vi "SECoP_dataCreateSECoPstatus.vi"(8 "error in (no error)":errorcluster, 11 "DLL path (in)":T2) -> (0 "error out":errorcluster, 2 "SECoP_dataPtr (out)":T1 {"ptr64" format="%.0x"; "ptr32" format="%.0x"}, 3 "DLL path (out)":T2)   [LabVIEW 2023, in "SECoP.lvlib"]
doc: "Call <b>\"SECoP_dataCreateSECoPstatus.vi\"</b> to create a basic data type for a SECoP status with IDLE/100 only. Use <b>\"SECoP_dataPutEnumeration.vi\"</b> to extend it. Free resources after use with <b>\"SECoP_dataDestroy.vi\"</b>.\nNote: You could also use </b>\"SECoP-addStatusParameter.vi\"</b> to get a similar result.\n\n<b>DLL path</b> input and output of cluster from \"SECoP-Initialize.vi\"\n<b>SECoP_dataPtr</b> created data"
uses:
  SECoP.lvlib
  SECoP-libraries.ctl
  SECoP-data.ctl
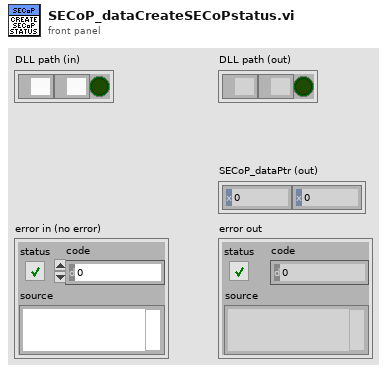
[diagram p1: front panel]
types:
  T1 = typedef "SECoP.lvlib/SECoP-data.ctl" = cluster{"ptr32":u32, "ptr64":u64}
  T2 = typedef "SECoP.lvlib/SECoP-libraries.ctl" = cluster{"serverDLL":path, "variantDLL":path, "cleanup_mode":bool}
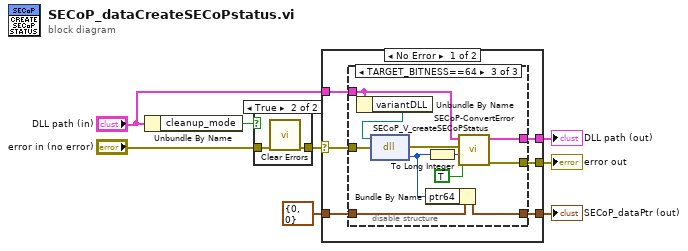
[diagram p0: block diagram]
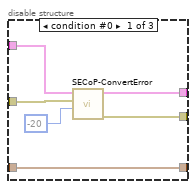
[diagram p3: hidden frame]
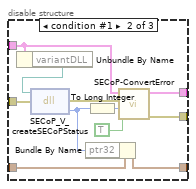
[diagram p4: hidden frame]
diagram:
  n1 = Unbundle By Name("DLL path (in)") -> ("cleanup_mode"=w6:bool)
  n2 = case shown="True" w6 {
    tunnel: "error in (no error)" -> [w9 w11]
    tunnel: [w9 w10] -> w4
    frame False {
    }
    frame True {
      n3 = call <vilib>:"Clear Errors.vi"("error in (no error)"=w11) -> ("error out"=w10:errorcluster)  [unwired: 5 in, 1 out]
    }
  }
  n4 = case shown="No Error" w4 {
    selector: w4 -> [w17 w47]
    tunnel: "DLL path (in)" -> [w16 w48]
    tunnel: [w14 w48] -> w8
    tunnel: [w15 w47] -> w7
    tunnel: [w12 w46] -> w3
    tunnel: T1 {"ptr32"=0, "ptr64"=0} ("SECoP_dataPtr (out)") -> [w13 w46]
    frame No Error {
      n5 = disable-structure shown="TARGET_BITNESS==64" {
        disable-tunnel: w17 -> [w23 w34 w45]
        disable-tunnel: w16 -> [w22 w25 w36]
        disable-tunnel: [w20 w30 w41] -> w15
        disable-tunnel: [w21 w29 w40] -> w14
        disable-tunnel: w13 -> [w18 w32 w43]
        disable-tunnel: [w18 w33 w44] -> w12
        frame condition #0 {
          n6 = call "SECoP-ConvertError.vi"("return code"=-20, "error in (no error)"=w23, "DLL path (in)"=w22) -> ("error out"=w20:errorcluster, "DLL path (out)"=w21:T2)  [unwired: 7 in]
        }
        frame condition #1 {
          n7 = Unbundle By Name(w25) -> ("variantDLL"=w24:path)
          n8 = dll-call lib="Z:/Praktische_Aufgaben/SECoP-LabVIEW2015/32bit/SECoP32.dll" fn="SECoP_V_createSECoPStatus"(path in=w24, error in=w34) -> (error out=w31:errorcluster, "return type"=w28:u32)  [unwired: 1 in, 1 out]
          n9 = Bundle By Name(cluster=w32, "ptr32"=w28) -> (w33:T1)
          n10 = To Long Integer(number=w28) -> (32bit integer=w26:i32)
          n11 = call "SECoP-ConvertError.vi"("return is boolean"=TRUE, "return code"=w26, "error in (no error)"=w31, "DLL path (in)"=w25) -> ("error out"=w30:errorcluster, "DLL path (out)"=w29:T2)  [unwired: 6 in]
        }
        frame condition #2 (active) {
          n12 = Unbundle By Name(w36) -> ("variantDLL"=w35:path)
          n13 = dll-call lib="Z:/Praktische_Aufgaben/SECoP-LabVIEW2015/32bit/SECoP32.dll" fn=" SECoP_V_createSECoPStatus" label="SECoP_V_createSECoPStatus"(path in=w35, error in=w45) -> (error out=w42:errorcluster, "return type"=w39:u64)  [unwired: 1 in, 1 out]
          n14 = Bundle By Name(cluster=w43, "ptr64"=w39) -> (w44:T1)
          n15 = To Long Integer(number=w39) -> (32bit integer=w37:i32)
          n16 = call "SECoP-ConvertError.vi"("return is boolean"=TRUE, "return code"=w37, "error in (no error)"=w42, "DLL path (in)"=w36) -> ("error out"=w41:errorcluster, "DLL path (out)"=w40:T2)  [unwired: 6 in]
        }
      }
    }
    frame Error {
    }
  }
  "DLL path (out)" <- w8
  "error out" <- w7
  "SECoP_dataPtr (out)" <- w3
